vi "GetVolumeInformation.vi"(0 "RootPathName (C:\\)":string="c:\\", 11 "error in (no error)":errorcluster) -> (1 "VolumeName":string, 2 "FileSystemName":string, 3 "VolumeSerialNumber":u32 format="%.0x", 4 "Dup Root Path name (C:\\)":string="c:\\", 6 "MaximumFile Name Length":u32, 10 "FileSystemFlags":u32, 15 "error out":errorcluster)   [LabVIEW 2018]
doc: "Uses an API call to retrieves the Volume Information for the requested drive.\nThe volume information incudes...\n\nThe name of the drive\nA unique identifier/serial number\nThe maximum filename length\nTthe type of file system (FAT, FAT32, NTFS. CDFS)\nFile System Flags\nThe File System Flags can be any combination of the following flags, with one exception: FS_FILE_COMPRESSION and FS_VOL_IS_COMPRESSED are mutually exclusive. \n\nFS_CASE_IS_PRESERVED If this flag is set, the file system preserves the case of filenames when it places a name on disk.\n\nFS_CASE_SENSITIVE If this flag is set, the file system supports case-sensitive filenames.\n\nFS_UNICODE_STORED_ON_DISK If this flag is set, the file system supports Unicode in filenames as they appear on disk.\n\nFS_PERSISTENT_ACLS If this flag is set, the file system preserves and enforces ACLs. For example, NTFS preserves and enforces ACLs, HPFS and FAT do not. \n\nFS_FILE_COMPRESSION The file system supports file-based compression.\n\nFS_VOL_IS_COMPRESSED The specified volume is a compressed volume; for example, a DoubleSpace volume."
uses:
  kernel32.dll
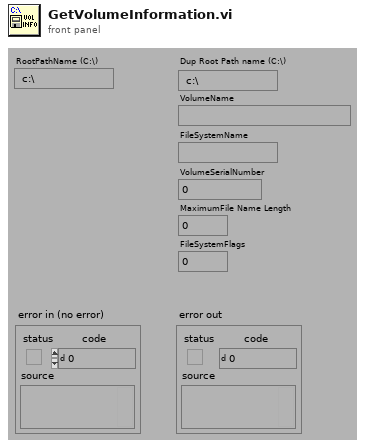
[diagram p1: front panel]
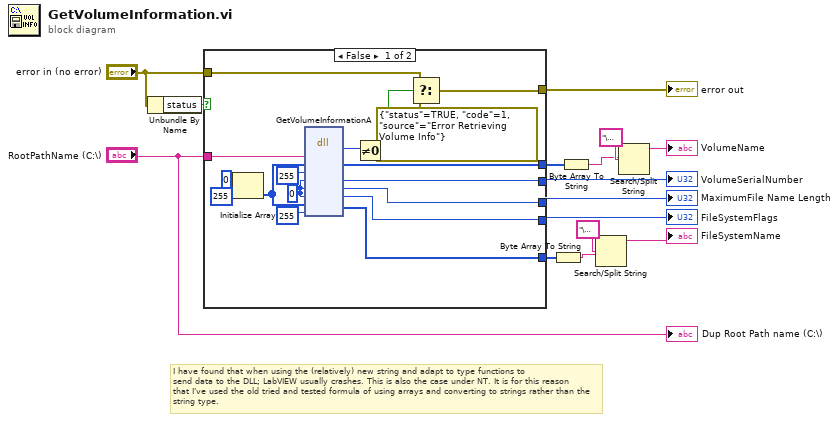
[diagram p0: block diagram]
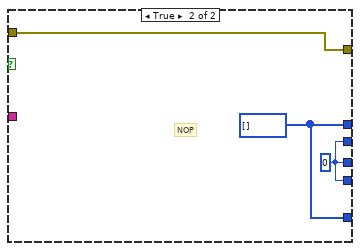
[diagram p2: hidden frame]
diagram:
  # "I have found that when using the (relatively) new string and adapt to type functions to\nsend data to the DLL; LabVIEW usually crashes. This is also the case under NT. It is for this reason\nthat I've used the old tried and tested formula of using arrays and converting to strings rather than the\nstring type."
  n1 = Unbundle By Name("error in (no error)") -> ("status"=w10:bool)
  n2 = case shown="False" w10 {
    tunnel: [w32 w34] -> w15
    tunnel: [w31 w34] -> w14
    tunnel: [w30 w34] -> w13
    tunnel: [w16 w33] -> w8
    tunnel: [w26 w33] -> w12
    tunnel: "RootPathName (C:\\)" -> [w25 _]
    tunnel: "error in (no error)" -> [w22 w35]
    tunnel: [w21 w35] -> w9
    frame False {
      w28 = u32 0 ("lpRootPathName")
      n3 = Initialize Array(u8 0, 255) -> (w19:u8[])
      n4 = dll-call lib="kernel32.dll" fn="GetVolumeInformationA" label="Get VolumeInformation"("lpRootPathName"=w25, "lpVolumeNameBuffer"=w19, "nVolumeNameSize"=u32 255, "lpVolumeSerialNumber"=w28, "lpMaximumComponentLength"=w28, "lpFileSystemFlags"=w28, "lpFileSystemNameBuffer"=w19, "nFileSystemNameSize"=u32 255) -> (w24:u8, "lpVolumeNameBuffer"=w26:u8[], "lpVolumeSerialNumber"=w32:u32, "lpMaximumComponentLength"=w31:u32, "lpFileSystemFlags"=w30:u32, "lpFileSystemNameBuffer"=w16:u8[])  [unwired: 6 in, 2 out]
      n5 = Not Equal To 0?(x=w24) -> (x != 0?=w23:bool)
      n6 = Select(t=w22, s=w23, f=errorcluster {"status"=TRUE, "code"=1, "source"="Error Retrieving Volume Info"}) -> (s? t:f=w21:errorcluster)
    }
    frame True {
      w33 = u8[] [] ("lpVolumeNameBuffer")
      w34 = u32 0 ("lpVolumeSerialNumber")
      # "NOP"
    }
  }
  "VolumeSerialNumber" <- w15
  "MaximumFile Name Length" <- w14
  "FileSystemFlags" <- w13
  "error out" <- w9
  n7 = Byte Array To String(unsigned byte array=w8) -> (string=w7:string)
  n8 = Byte Array To String(unsigned byte array=w12) -> (string=w3:string)
  n9 = Search/Split String(string=w7, search string/char (-)="\u0000" ("search char (-)")) -> (substring before match=→"FileSystemName":string)  [unwired: 3 out]
  n10 = Search/Split String(string=w3, search string/char (-)="\u0000" ("search char (-)")) -> (substring before match=→"VolumeName":string)  [unwired: 3 out]
  "Dup Root Path name (C:\\)" <- "RootPathName (C:\\)"
